vi "Analyze Frequency Response of Filter with Log Spaced Frequency Bins.vi"() -> ()   [LabVIEW 2023]
doc: "Demonstrates how to use the Filter Analysis VIs to analyze the frequency response of the designed filter with log spaced frequency bins.\n\nComplete the following steps to use this VI.\n1) Run the VI.\n2) Observe the plots on the Linear-Spaced Frequency Bins and Log-Spaced Frequency Bins graphs. Observe the different responses at the low frequency points from 0.1 Hz to 1 Hz.\n3) Examine the block diagram to learn how to get the log-spaced frequency response."
uses:
  <vilib>/addons/Digital Filter Design/_LpNorm.llb/dfd_Lp Norm Filter Type.ctl
  <vilib>/addons/Digital Filter Design/_Objects.llb/DFD Plot Settings.ctl
  <vilib>/addons/Digital Filter Design/Design.llb/DFD Least Pth Norm Design by Newton.vi
  <vilib>/addons/Digital Filter Design/Analysis.llb/DFD Plot Freq Response (Linear-Spaced).vi
  <vilib>/addons/Digital Filter Design/Analysis.llb/DFD Plot Freq Response (Frequency Vector).vi
  <vilib>/addons/Digital Filter Design/Analysis.llb/DFD Plot Freq Response (Log-Spaced).vi
  <vilib>/addons/Digital Filter Design/NI_DigFilterLicensed.lvlib
panel:
  out "Log-Spaced Frequency Bins":T1(graph)
  out "Linear-Spaced Frequency Bins":cluster{"f0":dbl, "df":dbl, "values":dbl[]}[](graph)
  in  "Band Specifications":T2(array[cluster])=[{"frequency point"=[{"frequency"=0.1, "magnitude"=0.031224824062232707, "weight"=1.0, "phase"=0.0}, {"frequency"=0.125, "magnitude"=0.04864072056914614, "weight"=1.0, "phase"=0.0}, {"frequency"=0.16, "magnitude"=0.07897688493998856, "weight"=1.0, "phase"=0.0}, {"frequency"=0.2, "magnitude"=0.12119926887749231, "weight"=1.0, "phase"=0.0}, {"frequency"=0.25, "magnitude"=0.18176070560954993, "weight"=1.0, "phase"=0.0}, {"frequency"=0.315, "magnitude"=0.2630267991895382, "weight"=1.0, "phase"=0.0}, {"frequency"=0.4, "magnitude"=0.35196542252476576, "weight"=1.0, "phase"=0.0}, {"frequency"=0.5, "magnitude"=0.4183116886514955, "weight"=1.0, "phase"=0.0}, {"frequency"=0.63, "magnitude"=0.45866964579820146, "weight"=1.0, "phase"=0.0}, {"frequency"=0.8, "magnitude"=0.47697981411922147, "weight"=1.0, "phase"=0.0}, {"frequency"=1.0, "magnitude"=0.4825029800597099, "weight"=1.0, "phase"=0.0}, {"frequency"=1.25, "magnitude"=0.48473011262436616, "weight"=1.0, "phase"=0.0}, {"frequency"=1.6, "magnitude"=0.49431068698683545, "weight"=1.0, "phase"=0.0}, {"frequency"=2.0, "magnitude"=0.5314959995066479, "weight"=1.0, "phase"=0.0}, {"frequency"=2.5, "magnitude"=0.6302313459908515, "weight"=1.0, "phase"=0.0}, {"frequency"=3.15, "magnitude"=0.8035261221856173, "weight"=1.0, "phase"=0.0}, {"frequency"=4.0, "magnitude"=0.9671637266500186, "weight"=1.0, "phase"=0.0}, {"frequency"=5.0, "magnitude"=1.0387236024226219, "weight"=1.0, "phase"=0.0}, {"frequency"=6.3, "magnitude"=1.0543868963912588, "weight"=1.0, "phase"=0.0}, {"frequency"=8.0, "magnitude"=1.0363346044310422, "weight"=1.0, "phase"=0.0}, {"frequency"=10.0, "magnitude"=0.9885530946569389, "weight"=1.0, "phase"=0.0}, {"frequency"=12.5, "magnitude"=0.9026097074709752, "weight"=1.0, "phase"=0.0}, {"frequency"=16.0, "magnitude"=0.7691304402866096, "weight"=1.0, "phase"=0.0}, {"frequency"=20.0, "magnitude"=0.6360628048372603, "weight"=1.0, "phase"=0.0}, {"frequency"=25.0, "magnitude"=0.5128613839913648, "weight"=1.0, "phase"=0.0}, {"frequency"=31.5, "magnitude"=0.4031809464434653, "weight"=1.0, "phase"=0.0}, {"frequency"=40.0, "magnitude"=0.31441264202587954, "weight"=1.0, "phase"=0.0}, {"frequency"=50.0, "magnitude"=0.24575366312150465, "weight"=1.0, "phase"=0.0}, {"frequency"=63.0, "magnitude"=0.18599445632225764, "weight"=1.0, "phase"=0.0}, {"frequency"=80.0, "magnitude"=0.1324341535194665, "weight"=1.0, "phase"=0.0}, {"frequency"=100.0, "magnitude"=0.08871560120379608, "weight"=1.0, "phase"=0.0}, {"frequency"=125.0, "magnitude"=0.05401321147646348, "weight"=1.0, "phase"=0.0}, {"frequency"=160.0, "magnitude"=0.028477378001737455, "weight"=1.0, "phase"=0.0}, {"frequency"=200.0, "magnitude"=0.01517050367459336, "weight"=1.0, "phase"=0.0}, {"frequency"=250.0, "magnitude"=0.007906786279998253, "weight"=1.0, "phase"=0.0}, {"frequency"=315.0, "magnitude"=0.003981071705534973, "weight"=1.0, "phase"=0.0}, {"frequency"=400.0, "magnitude"=0.0019498445997580456, "weight"=1.0, "phase"=0.0}]}] {"frequency point"."weight" format="%.2f"}
  # "Select Help>>Show Context Help and move the cursor over the VI icon for more information."
  # "freq"
  # "magnitude"
  # "weight"
  # "phase"
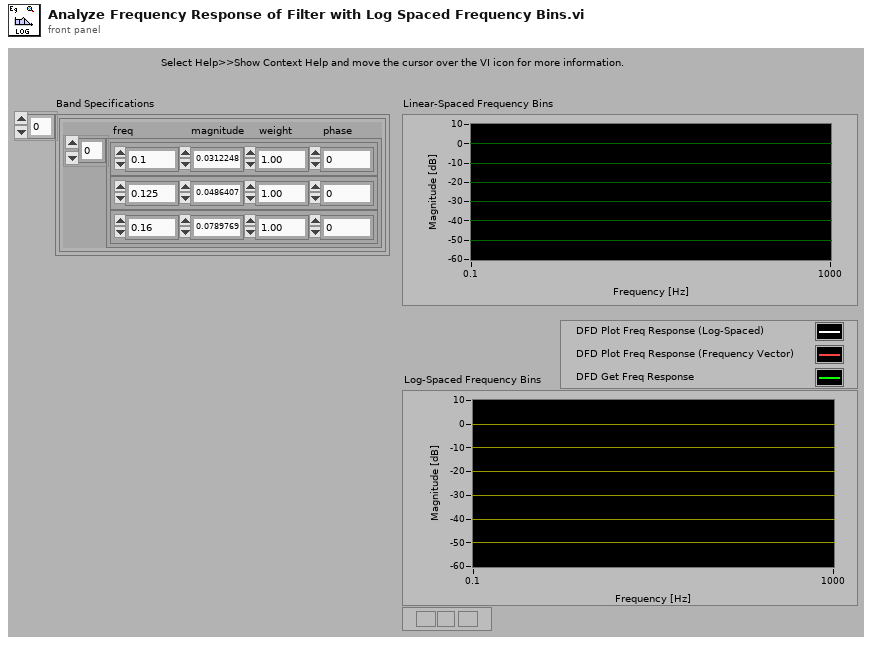
[diagram p1: front panel]
types:
  T1 = cluster{"freq points":dbl[], "magnitude":dbl[]}[]
  T2 = cluster{"frequency point":cluster{"frequency":dbl, "magnitude":dbl, "weight":dbl, "phase":dbl}[]}[]
  T3 = typedef "NI_DigFilterLicensed.lvlib/DFD Plot Settings.ctl" = cluster{"# freq bins":i32, "low frequency [Hz]":dbl, "high frequency [Hz]":dbl}
  T4 = typedef "NI_DigFilterLicensed.lvlib/dfd_Lp Norm Filter Type.ctl" = enum16{"Symmetric", "Antisymmetric", "Differentiator", "Hilbert", "Minimum Phase", "Maximum Phase"}
  T5 = typedef "NI_DigFilterLicensed.lvlib/DFD Filter Obj.ctl" = cluster{"mSRate_Fs":dbl, "mSRate_Version":string, "mSRate_Comments":string, "mSRate_OrgCoef":T6, "mSRate_CurCoef":T6, "mSRate_Quantized?":bool, "mSRate_QCoef":T6, "mSRate_QSettings":T8[], "mSRate_Order":i32, "mSRate_Scaling":cluster{"mSRate_ScaleByPowerOf2?":bool, "mSRate_ScaleType":T10}}
  T6 = typedef "NI_DigFilterLicensed.lvlib/DFD Filter Coef.ctl" = cluster{"type":T7, "gain":dbl, "coef a (k)":dbl[], "coef b (v)":dbl[]}
  T7 = typedef "NI_DigFilterLicensed.lvlib/DFD Filter Structure Type Selector.ctl" = enum16{"Undefined", "FIR Direct Form", "FIR Direct Form Transposed", "FIR Symmetric", "FIR Antisymmetric", "IIR Direct Form I", "IIR Direct Form I Transposed", "IIR Direct Form II", "IIR Direct Form II Transposed", "IIR Cascaded Second Order Sections Form I", "IIR Cascaded Second Order Sections Form I Transposed", "IIR Cascaded Second Order Sections Form II", "IIR Cascaded Second Order Sections Form II Transposed", "Lattice Allpass (basic sections)", "Lattice Allpass (one multiplier sections)", "Lattice Allpass (normalized sections)", "Lattice AR (basic sections)", "Lattice AR (one multiplier sections)", "Lattice AR (normalized sections)", "Lattice MA (minimum phase)", "Lattice MA (maximum phase)", "Lattice ARMA (basic sections)", "Lattice ARMA (one multiplier sections)", "Lattice ARMA (normalized sections)"}
  T8 = typedef "NI_DigFilterLicensed.lvlib/dfd_Internal Quantization Settings.ctl" = cluster{"source":T9, "wl":i16, "iwl":i16, "overflow mode":enum16{"Saturation", "Wrap"}, "rounding mode":enum16{"Nearest", "Truncation"}, "signed?":bool}
  T9 = typedef "NI_DigFilterLicensed.lvlib/dfd_Internal Quantization Srcs.ctl" = u16
  T10 = typedef "NI_DigFilterLicensed.lvlib/DFD Coef Norm Type.ctl" = enum16{"No Norm", "Time Domain 1-Norm", "Time Domain 2-Norm", "Time Domain Inf-Norm"}
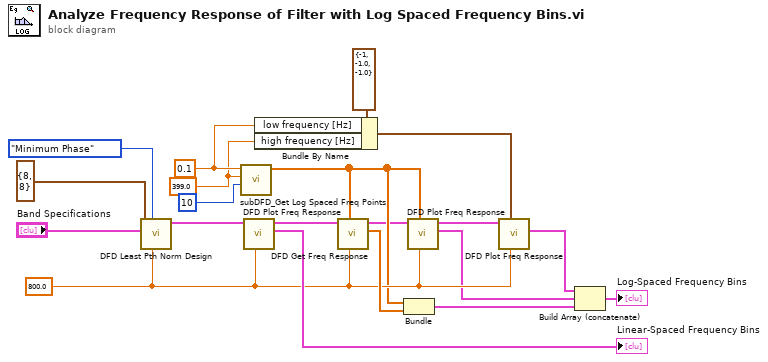
[diagram p0: block diagram]
diagram:
  w10 = 399.0 ("end frequency point")
  w11 = 0.1 ("start frequency point")
  w8 = 800.0 ("fs [Hz]")
  n1 = call-poly <vilib>:"DFD Least Pth Norm Design.vi"("fs [Hz]"=w8, "filter type"=dfd_Lp_Norm_Filter_Type."Minimum Phase" ("Filter Type"), "band specs"="Band Specifications", "order"=cluster{"num":i32, "den":i32} {"num"=8, "den"=8} ("Order")) -> ("filter out"=w17:T5)  [unwired: 4 in, 3 out]
  n2 = call <vilib>:"subDFD_Get Log Spaced Freq Points.vi"("# points per log freq bin"=10 ("# points per log frequency bin"), "end frequency point"=w10, "start frequency point"=w11) -> ("freq points"=w7:dbl[])  [unwired: 8 out]
  n3 = call-poly <vilib>:"DFD Plot Freq Response.vi"("fs [Hz]"=w8, "filter in"=w17) -> ("magnitude response"=→"Linear-Spaced Frequency Bins":cluster{"f0":dbl, "df":dbl, "values":dbl[]}[], "filter out"=w6:T5)  [unwired: 6 in, 2 out]
  n4 = Bundle By Name(cluster=T3 {"# freq bins"=-1, "low frequency [Hz]"=-1.0, "high frequency [Hz]"=-1.0} ("plot settings"), "low frequency [Hz]"=w11, "high frequency [Hz]"=w10) -> (w9:T3)
  n5 = call <vilib>:"DFD Get Freq Response.vi"("fs [Hz]"=w8, "freq points [Hz]"=w7, "filter in"=w6) -> ("magnitude"=w16:dbl[], "filter out"=w5:T5)  [unwired: 4 in, 3 out]
  n6 = Bundle("freq points"=w7, "magnitude"=w16) -> (w3:cluster{"freq points":dbl[], "magnitude":dbl[]})  [unwired: 1 out]
  n7 = call-poly <vilib>:"DFD Plot Freq Response.vi"("fs [Hz]"=w8, "frequency vector [Hz]"=w7, "filter in"=w5) -> ("magnitude response"=w2:cluster{"bins":dbl[], "response FXP":dbl[]}[], "filter out"=w4:T5)  [unwired: 5 in, 2 out]
  n8 = call-poly <vilib>:"DFD Plot Freq Response.vi"("fs [Hz]"=w8, "plot settings"=w9, "filter in"=w4) -> ("magnitude response"=w1:cluster{"bins":dbl[], "response FXP":dbl[]}[])  [unwired: 5 in, 3 out]
  n9 = Build Array (concatenate)(w1, w2, w3) -> (→"Log-Spaced Frequency Bins":T1)
